vi "Vehicle control.vi"() -> ()   [LabVIEW 2020]
panel:
  in  "stop":bool
  in  "SPEED CONTROL REVERSE":dbl(knob) scale=0.0..100.0
  in  "SPEED CONTROL FORWARD":dbl(knob) scale=0.0..100.0
  in  "Slide":dbl(slide) scale=0.0..100.0
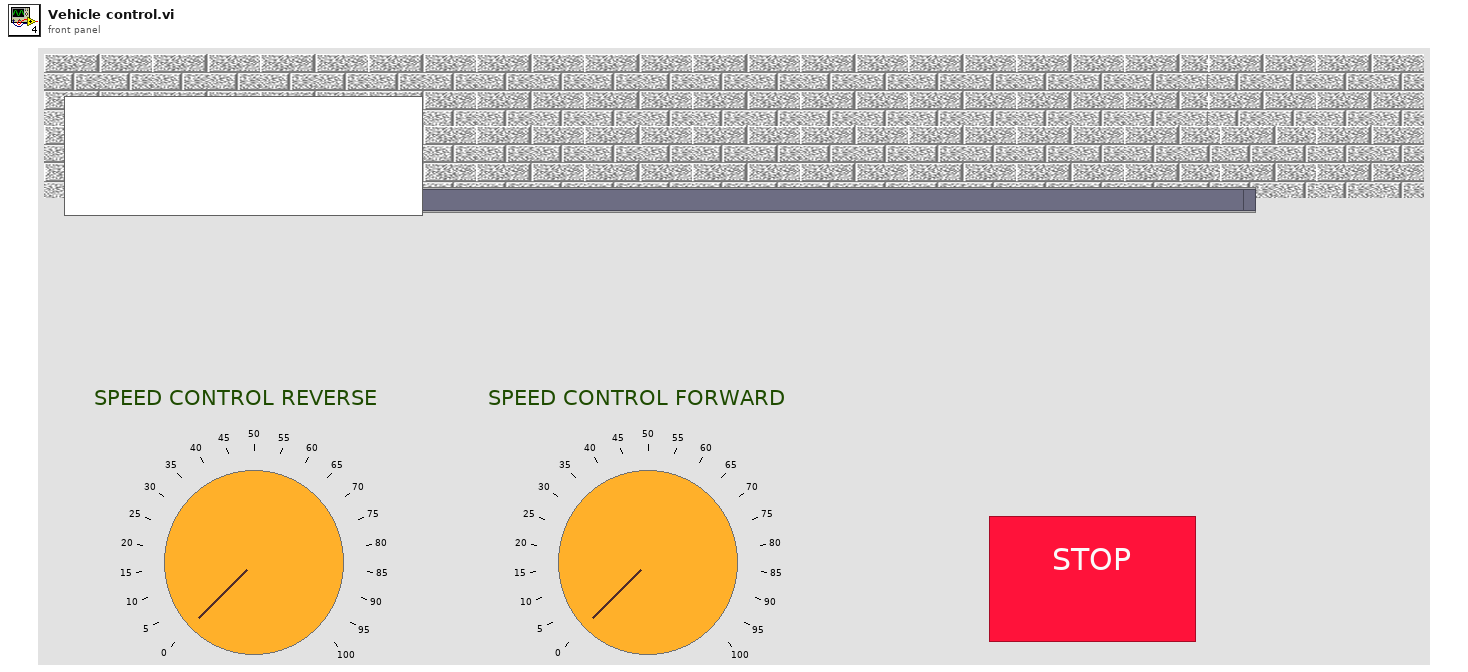
[diagram p1: front panel]
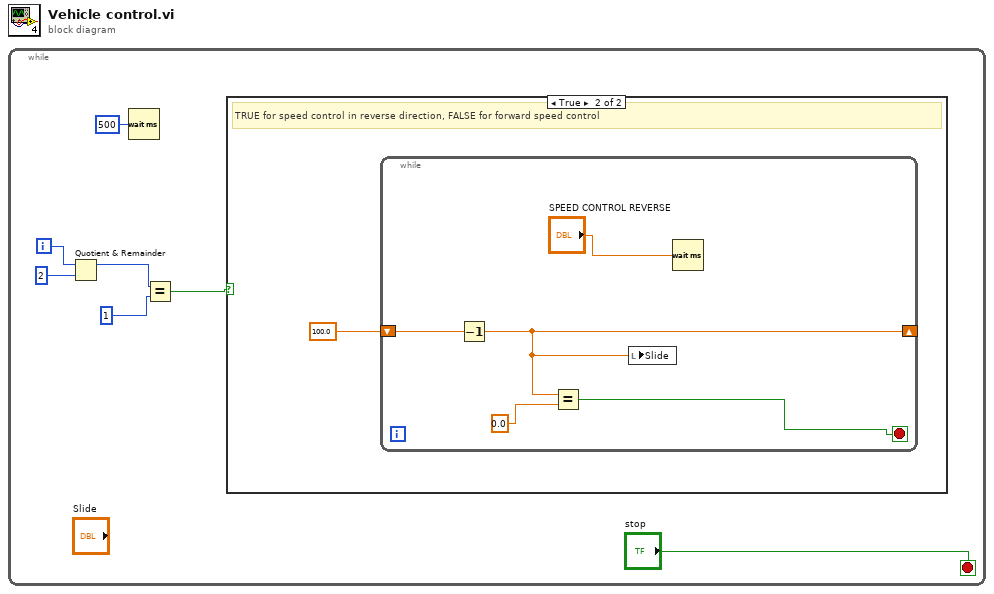
[diagram p0: block diagram]
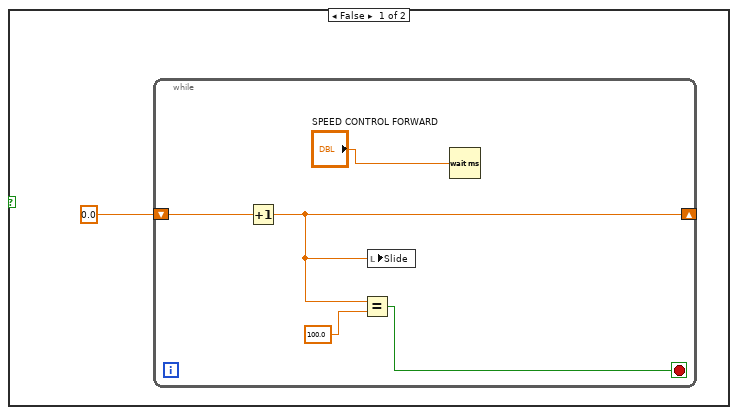
[diagram p2: hidden frame]
diagram:
  n1 = while {
    i -> [w5]
    stop <- "stop" stop-if-true
    n2 = Quotient & Remainder(x=w5, y=2) -> (x-y*floor(x/y)=w4:i32)  [unwired: 1 out]
    n3 = Wait (ms)(milliseconds to wait=u32 500) -> ()  [unwired: 1 out]
    n4 = Equal?(x=w4, y=1) -> (x = y?=w2:bool)
    n5 = case shown="True" w2 {
      frame False {
        n6 = while {
          shift-right: [w9] -> _
          shift-left: 0.0 -> [w13]
          stop <- w11 stop-if-true
          n7 = Increment(x=w13) -> (x+1=w9:dbl)
          n8 = Equal?(x=w9, y=100.0) -> (x = y?=w11:bool)
          n9 = local write "Slide"(w9) -> ()
          n10 = Wait (ms)(milliseconds to wait="SPEED CONTROL FORWARD") -> ()  [unwired: 1 out]
        }
      }
      frame True {
        # "TRUE for speed control in reverse direction, FALSE for forward speed control"
        n11 = while {
          shift-right: [w16] -> _
          shift-left: 100.0 -> [w17]
          stop <- w18 stop-if-true
          n12 = Decrement(x=w17) -> (x-1=w16:dbl)
          n13 = Equal?(x=w16, y=0.0) -> (x = y?=w18:bool)
          n14 = local write "Slide"(w16) -> ()
          n15 = Wait (ms)(milliseconds to wait="SPEED CONTROL REVERSE") -> ()  [unwired: 1 out]
        }
      }
    }
  }
